vi "correct_peak_detect.vi"(8 "plus-minus crossing?":bool[](array[boolean]), 9 "minus-plus crossing?":bool[](array[boolean]), 10 "Peak Amplitudes":dbl[](array[numeric]), 11 "Peak Locations":dbl[](array[numeric])) -> (2 "Corrected Peak Amplitudes":dbl[](array[numeric]), 3 "Corrected Peak Locations":dbl[](array[numeric]))   [LabVIEW 2020]
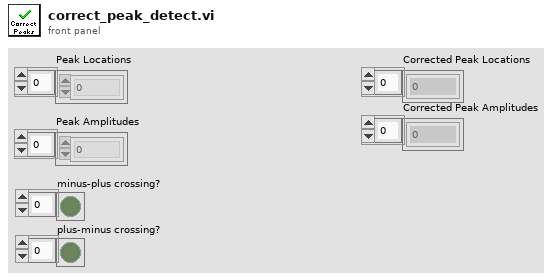
[diagram p1: front panel]
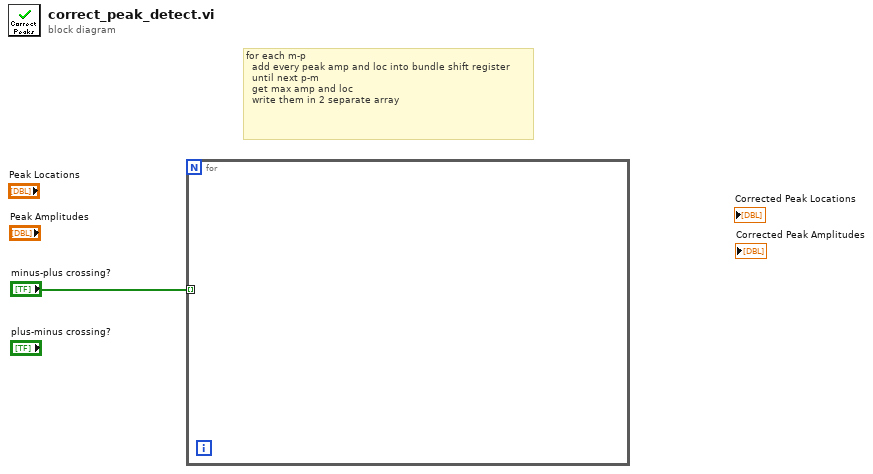
[diagram p0: block diagram]
diagram:
  # "for each m-p\n  add every peak amp and loc into bundle shift register\n  until next p-m\n  get max amp and loc\n  write them in 2 separate array"
  n1 = for {
    tunnel: "minus-plus crossing?" -> [_] mode=indexing
  }
